vi "Parse Text-Tag.vi"(8 "Error In":errorcluster) -> (0 "Error Out":errorcluster)   [LabVIEW 2017, in "Tests.lvlib" / "Parser.lvlib"]
uses:
  Parser.lvlib
  src/Mustache/Public/Tokens/Public/Text/Text.lvclass
  src/Mustache/Public/Tokens/Public/Tag/Tag.lvclass
  src/Mustache/Public/Tokens/Public/Tag/Tag.lvclass/Tag.ctl
  src/Mustache/Public/Readers/Public/String/String.lvclass
  D:/Users/cfield/Code/Field R&D Services/Mustache/feature-lv-original-parser/src/Mustache/Public/Readers/Public/Abstract/Abstract.lvclass
  <vilib>/addons/_JKI Toolkits/Caraya/classes/Test/Test.lvclass
  src/Mustache/Public/Parser/Parser.lvclass
  <vilib>/addons/_JKI Toolkits/Caraya/classes/Assert/Assert.lvclass
  src/Mustache/Public/Tokens/Public/Abstract/Abstract.lvclass
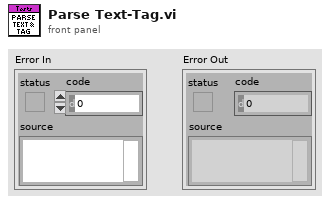
[diagram p1: front panel]
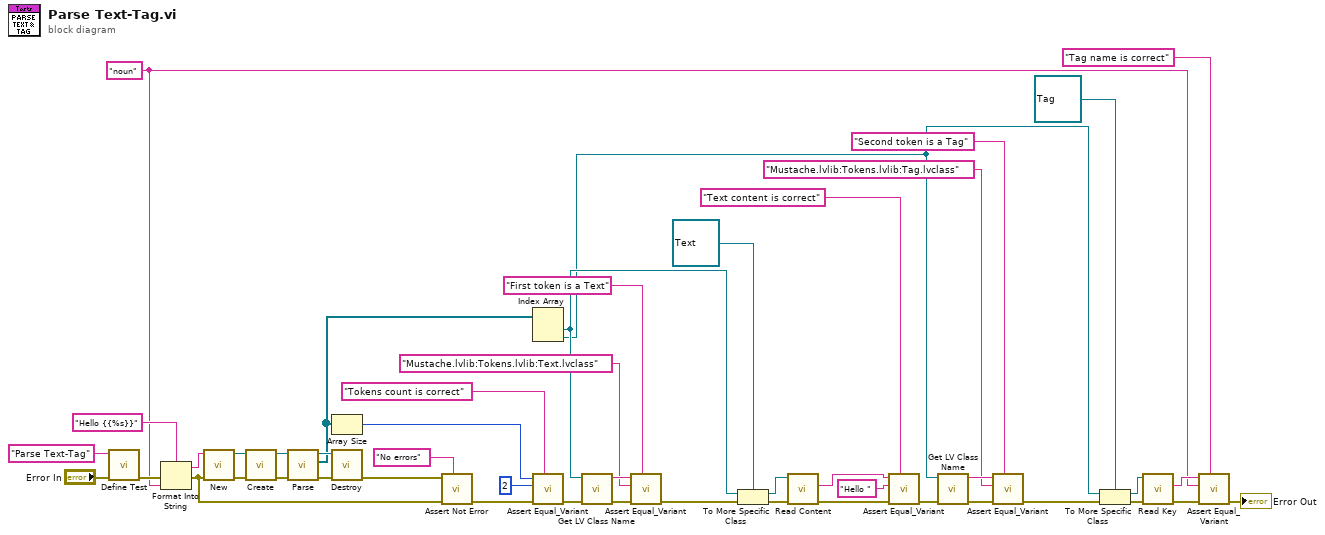
[diagram p0: block diagram]
diagram:
  w2 = "noun" ("String")
  n1 = call <vilib>:"Define Test.vi"("error in (no error)"="Error In", "Label (VI Title)"="Parse Text-Tag") -> ("error out"=w39:errorcluster)  [unwired: 9 in]
  n2 = Format Into String(format string="Hello {{%s}}", error in=w39, w2) -> (resulting string=w19:string, error out=w21:errorcluster)  [unwired: 1 in]
  n3 = call "New.vi"("Error In"=w21, "String"=w19) -> ("Error Out"=w45:errorcluster, "String"=w46:refnum<class "String.lvclass">)  [unwired: 8 in]
  n4 = call "Create.vi"("Error In"=w45, "Reader"=w46) -> ("Error Out"=w44:errorcluster, "Parser"=w43:refnum<class "Parser.lvclass">)  [unwired: 8 in]
  n5 = call "Parse.vi"("Error In"=w44, "Parser In"=w43) -> ("Error Out"=w41:errorcluster, "Tokens"=w32:refnum<class "Abstract.lvclass">[], "Parser Out"=w42:refnum<class "Parser.lvclass">)  [unwired: 7 in]
  n6 = Array Size(array=w32) -> (size(s)=w35:i32)
  n7 = call "Destroy.vi"("Error In"=w41, "Parser"=w42) -> ("Error Out"=w40:errorcluster)  [unwired: 9 in]
  n8 = call <vilib>:"Assert Not Error.vi"("Label"="No errors", "error in (no error)"=w21, "Not Error?"=w40) -> ("error out"=w37:errorcluster)  [unwired: 8 in]
  n9 = Index Array(array=w32) -> (element #1=w17:refnum<class "Abstract.lvclass">, element #2=w8:refnum<class "Abstract.lvclass">)  [unwired: 2 in]
  n10 = call <vilib>:"Assert Equal_Variant.vi"("Label"="Tokens count is correct", "error in (no error)"=w37, "Y"=2 ("size(s)"), "X"=w35) -> ("error out"=w33:errorcluster)  [unwired: 7 in]
  n11 = call <vilib>:"Get LV Class Name.vi"("error in (no error)"=w33, "object"=w17) -> ("error out"=w31:errorcluster, "class name"=w30:string)  [unwired: 8 in]
  n12 = call <vilib>:"Assert Equal_Variant.vi"("Label"="First token is a Text", "error in (no error)"=w31, "Y"="Mustache.lvlib:Tokens.lvlib:Text.lvclass", "X"=w30) -> ("error out"=w27:errorcluster)  [unwired: 7 in]
  n13 = To More Specific Class(target class=refnum<class "Text.lvclass"> refnum ("Mustache.lvlib:Tokens.lvlib:Text.lvclass"), reference=w17, error in=w27) -> (specific class reference=w14:refnum<class "Text.lvclass">, error out=w18:errorcluster)
  n14 = call "Read Content.vi"("Error In"=w18, "Text In"=w14) -> ("Error Out"=w15:errorcluster, "Content"=w12:string)  [unwired: 7 in, 1 out]
  n15 = call <vilib>:"Assert Equal_Variant.vi"("Label"="Text content is correct", "error in (no error)"=w15, "Y"="Hello ", "X"=w12) -> ("error out"=w13:errorcluster)  [unwired: 7 in]
  n16 = call <vilib>:"Get LV Class Name.vi"("error in (no error)"=w13, "object"=w8) -> ("error out"=w26:errorcluster, "class name"=w25:string)  [unwired: 8 in]
  n17 = call <vilib>:"Assert Equal_Variant.vi"("Label"="Second token is a Tag", "error in (no error)"=w26, "Y"="Mustache.lvlib:Tokens.lvlib:Tag.lvclass", "X"=w25) -> ("error out"=w23:errorcluster)  [unwired: 7 in]
  n18 = To More Specific Class(target class=refnum<class "Tag.lvclass"> refnum ("Mustache.lvlib:Tokens.lvlib:Tag.lvclass"), reference=w8, error in=w23) -> (specific class reference=w5:refnum<class "Tag.lvclass">, error out=w9:errorcluster)
  n19 = call "Read Key.vi"("Error In"=w9, "Tag In"=w5) -> ("Error Out"=w6:errorcluster, "Key"=w3:string)  [unwired: 7 in, 1 out]
  n20 = call <vilib>:"Assert Equal_Variant.vi"("Label"="Tag name is correct", "error in (no error)"=w6, "Y"=w2, "X"=w3) -> ("error out"=→"Error Out":errorcluster)  [unwired: 7 in]
